vi "Scaled Value To Raw.vi"(1 "Scaling Constants":T1, 2 "dbl Scaled Value":dbl) -> (7 "u16 Raw Value":u16 format="%4x")   [LabVIEW 2021]
uses:
  <vilib>/myRIO/Common/Instrument Driver Framework/Utilities/typedefs/Analog Scaling Constants.ctl
panel:
  # "Converts scaled dbl value to raw ADC u16 value based on the scaling constants."
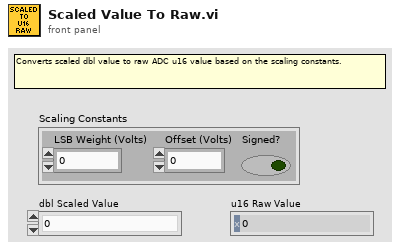
[diagram p1: front panel]
types:
  T1 = typedef "Analog Scaling Constants.ctl" = cluster{"LSB Weight (Volts)":dbl, "Offset (Volts)":dbl, "Signed?":bool}
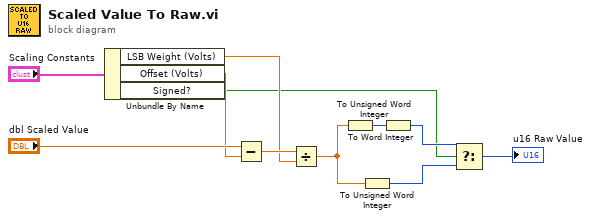
[diagram p0: block diagram]
diagram:
  n1 = Unbundle By Name("Scaling Constants") -> ("LSB Weight (Volts)"=w7:dbl, "Offset (Volts)"=w9:dbl, "Signed?"=w1:bool)
  n2 = Subtract(x="dbl Scaled Value", y=w9) -> (x-y=w8:dbl)
  n3 = Divide(x=w8, y=w7) -> (x/y=w6:dbl)
  n4 = To Word Integer(number=w6) -> (16bit integer=w5:i16)
  n5 = To Unsigned Word Integer(number=w6) -> (unsigned 16bit integer=w4:u16)
  n6 = To Unsigned Word Integer(number=w5) -> (unsigned 16bit integer=w3:u16)
  n7 = Select(t=w3, s=w1, f=w4) -> (s? t:f=→"u16 Raw Value":u16)
